vi "Pack Step Value.vi"(8 "error in":errorcluster, 10 "Value":string, 11 "Filter Step in":refnum<class "Filter Step.lvclass">) -> (0 "error out":errorcluster, 3 "Filter Step out":refnum<class "Filter Step.lvclass">)   [LabVIEW 2016, in "Controller.lvlib" / "Filter Step.lvclass"]
uses:
  Filter Step.lvclass
  Filter Step.lvclass/Filter Step.ctl
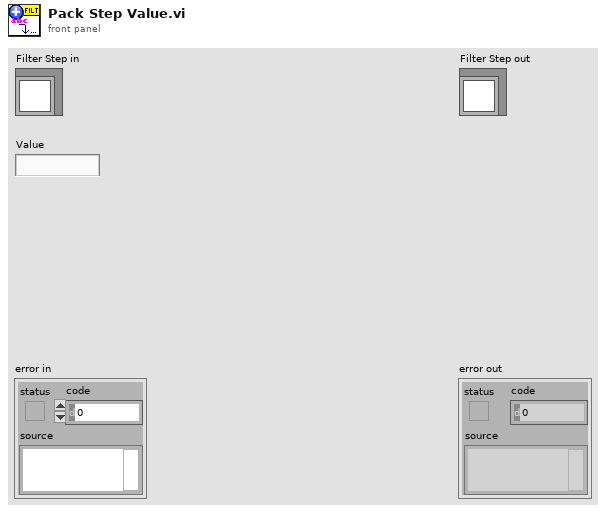
[diagram p1: front panel]
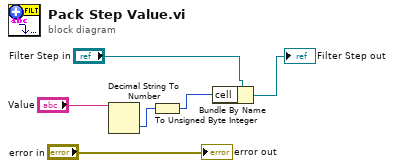
[diagram p0: block diagram]
diagram:
  n1 = Decimal String To Number(string="Value") -> (number=w2:i32)  [unwired: 2 in, 1 out]
  n2 = To Unsigned Byte Integer(number=w2) -> (unsigned 8bit integer=w1:u8)
  n3 = Bundle By Name(cluster="Filter Step in", "cell"=w1) -> (→"Filter Step out":refnum<class "Filter Step.lvclass">)
  "error out" <- "error in"
